vi "FGV REP.vi"(9 "Period of Excitation":string, 10 "Date/Time of Excitation":string, 11 "Enum":T1) -> (3 "Array":string[][](array[string]))   [LabVIEW 2014]
uses:
  set_get.ctl
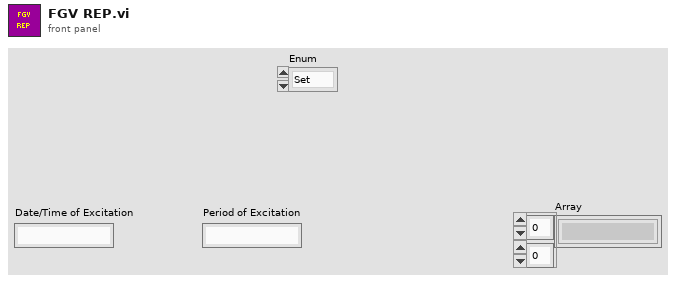
[diagram p1: front panel]
types:
  T1 = typedef "set_get.ctl" = enum16{"Set", "Get"}
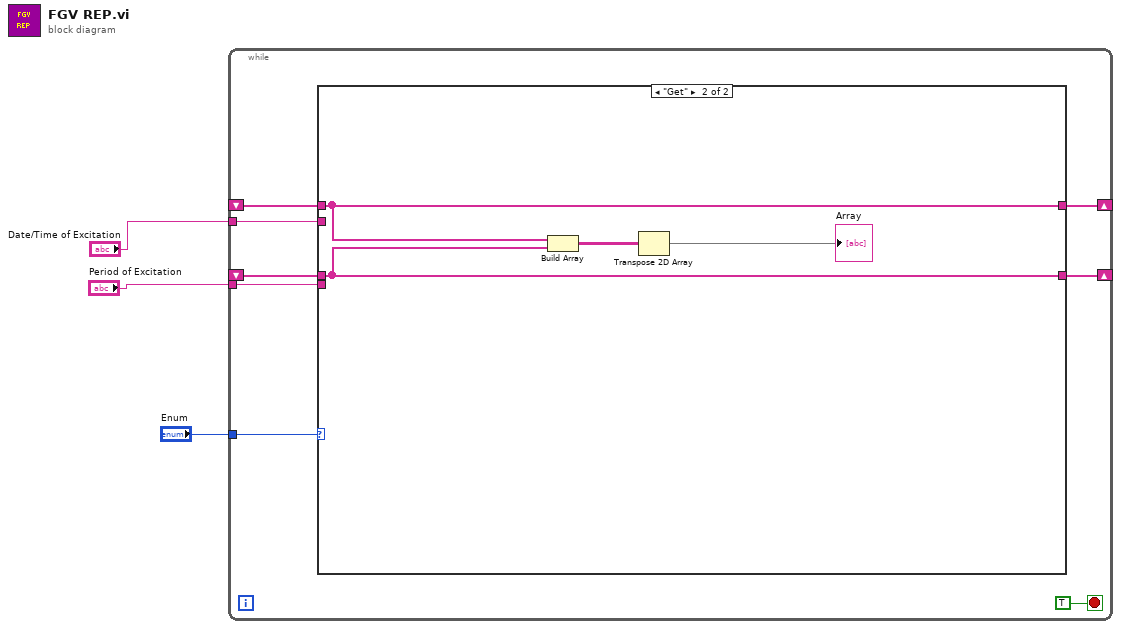
[diagram p0: block diagram]
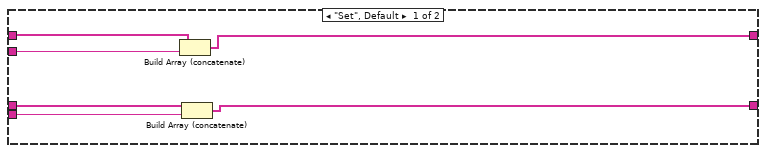
[diagram p2: hidden frame]
diagram:
  n1 = while {
    tunnel: "Enum" -> [w10]
    tunnel: "Date/Time of Excitation" -> [w9]
    tunnel: "Period of Excitation" -> [w8]
    shift-right: [w7] -> _
    shift-left: _ -> [w5]
    shift-right: [w6] -> _
    shift-left: _ -> [w4]
    stop <- TRUE stop-if-true
    n2 = case shown="\"Get\"" w10 {
      tunnel: w9 -> [w17 _]
      tunnel: w8 -> [w13 _]
      tunnel: [w14 w20] -> w7
      tunnel: [w12 w19] -> w6
      tunnel: w5 -> [w16 w20]
      tunnel: w4 -> [w15 w19]
      frame "Set", Default {
        n3 = Build Array (concatenate)(w16, w17) -> (w14:string[])
        n4 = Build Array (concatenate)(w15, w13) -> (w12:string[])
      }
      frame "Get" {
        n5 = Build Array(w20, w19) -> (w21:string[][])
        n6 = Transpose 2D Array(2D array=w21) -> (transposed array=→"Array":string[][])
      }
    }
  }
